vi "测试.vi"() -> ()   [LabVIEW 2014]
panel:
  in  "退出":bool
  in  "数组 2":T1(array[cluster])
  in  "簇":T2
  in  "数组":dbl[][](array[numeric])
  in  "组合框":string(combo)
  in  "字符串":string
  in  "布尔 2":bool
  in  "布尔":bool
  in  "数值1":dbl
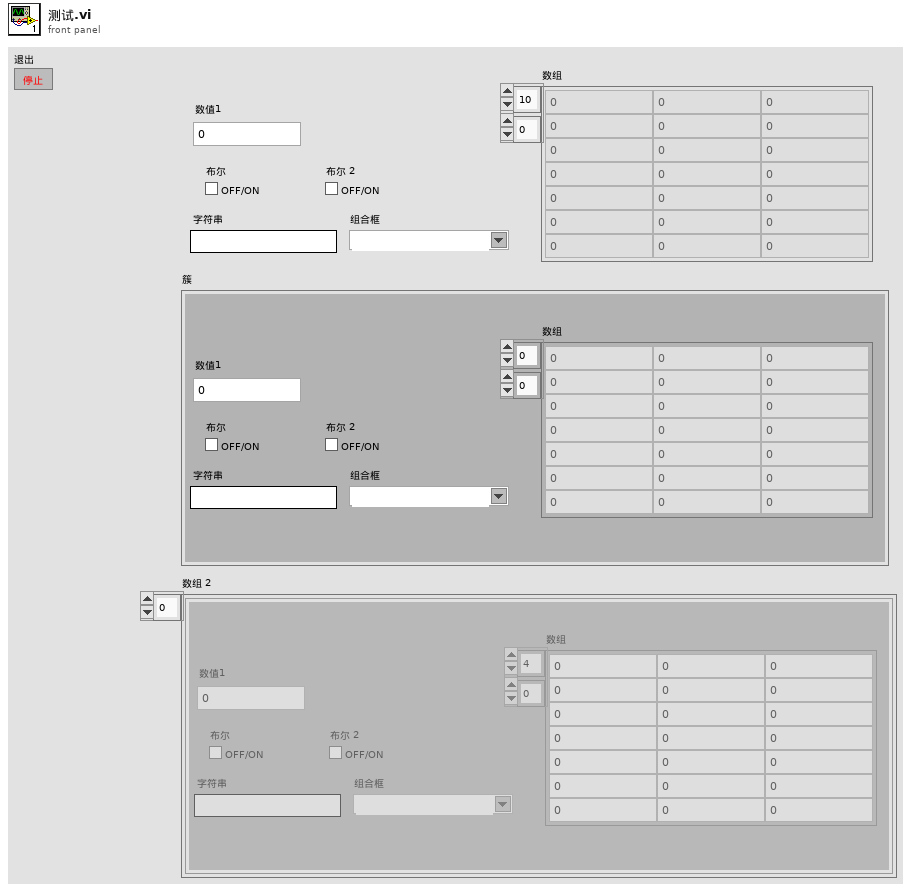
[diagram p1: front panel]
types:
  T1 = cluster{"数值1":dbl, "布尔":bool, "布尔 2":bool, "字符串":string, "组合框":string, "数组":dbl[][]}[]
  T2 = cluster{"数值1":dbl, "布尔":bool, "布尔 2":bool, "字符串":string, "组合框":string, "数组":dbl[][]}
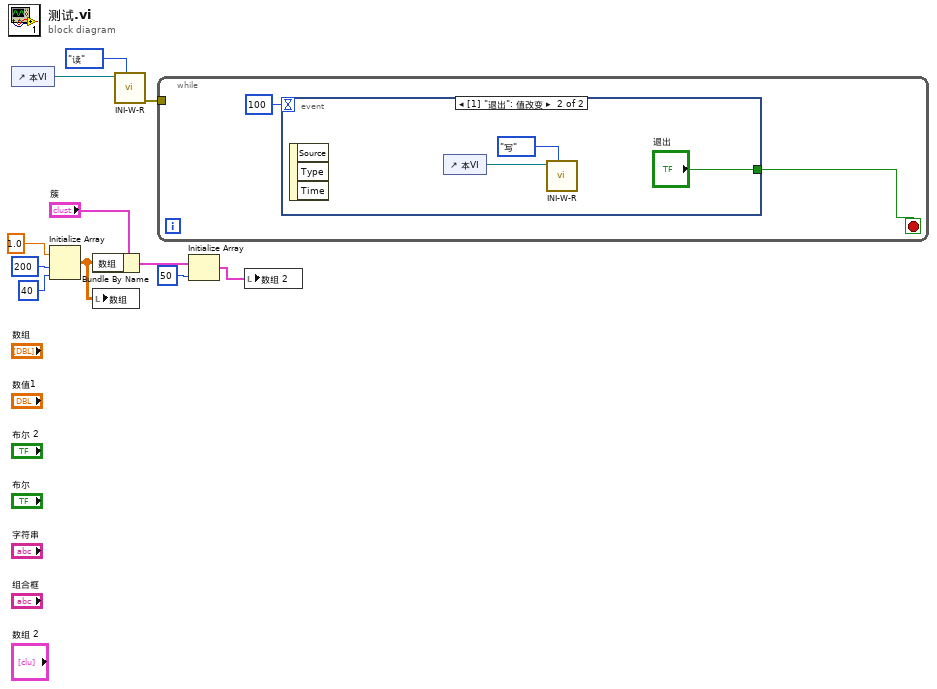
[diagram p0: block diagram]
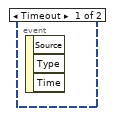
[diagram p2: hidden frame]
diagram:
  n1 = control-ref of="本VI"() -> (w3:refnum<vi>)
  n2 = Initialize Array(1.0 ("元素"), 200 ("维数大小"), 40 ("维数大小")) -> (w8:dbl[][])
  n3 = Bundle By Name(cluster="簇", "数组"=w8) -> (w7:T2)
  n4 = local write "数组"(w8) -> ()
  n5 = call "INI-W-R.vi"("W/R"=enum16{"读", "写"}."读", "VI ref"=w3) -> ("error out"=w2:errorcluster)  [unwired: 9 in]
  n6 = while {
    tunnel: w2 -> [_]
    stop <- w12 stop-if-true
    n7 = event shown="[1] \"退出\": 值改变" {
      selector: _ -> [_ _]
      dyn-events: _ -> [_ _]
      timeout: 100 -> [_ _]
      tunnel: [_ "退出"] -> w12
      event Timeout {
        n8 = event-data() -> ()  [unwired: 1 in, 3 out]
      }
      event "退出": Value Change {
        n9 = event-data() -> ()  [unwired: 1 in, 3 out]
        n10 = control-ref of="本VI"() -> (w15:refnum<vi>)
        n11 = call "INI-W-R.vi"("W/R"=enum16{"读", "写"}."写", "VI ref"=w15) -> ()  [unwired: 9 in, 1 out]
      }
    }
  }
  n12 = Initialize Array(w7, 50 ("维数大小")) -> (w1:T1)
  n13 = local write "数组 2"(w1) -> ()
